vi "CDS Library Load.vi"(8 "error in (no error)":errorcluster, 11 "DMA Channel Testing in":refnum<class "DMA Channel Testing.lvclass">) -> (0 "error out":errorcluster, 3 "DMA Channel Testing out":refnum<class "DMA Channel Testing.lvclass">)   [LabVIEW 2019, in "DMA Channel Testing.lvclass"]
uses:
  DMA Channel Testing.lvclass
  DMA Channel Testing.lvclass/DMA Channel Testing.ctl
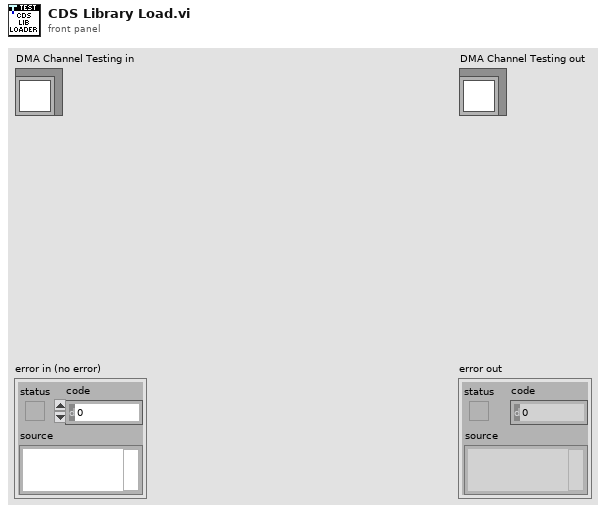
[diagram p1: front panel]
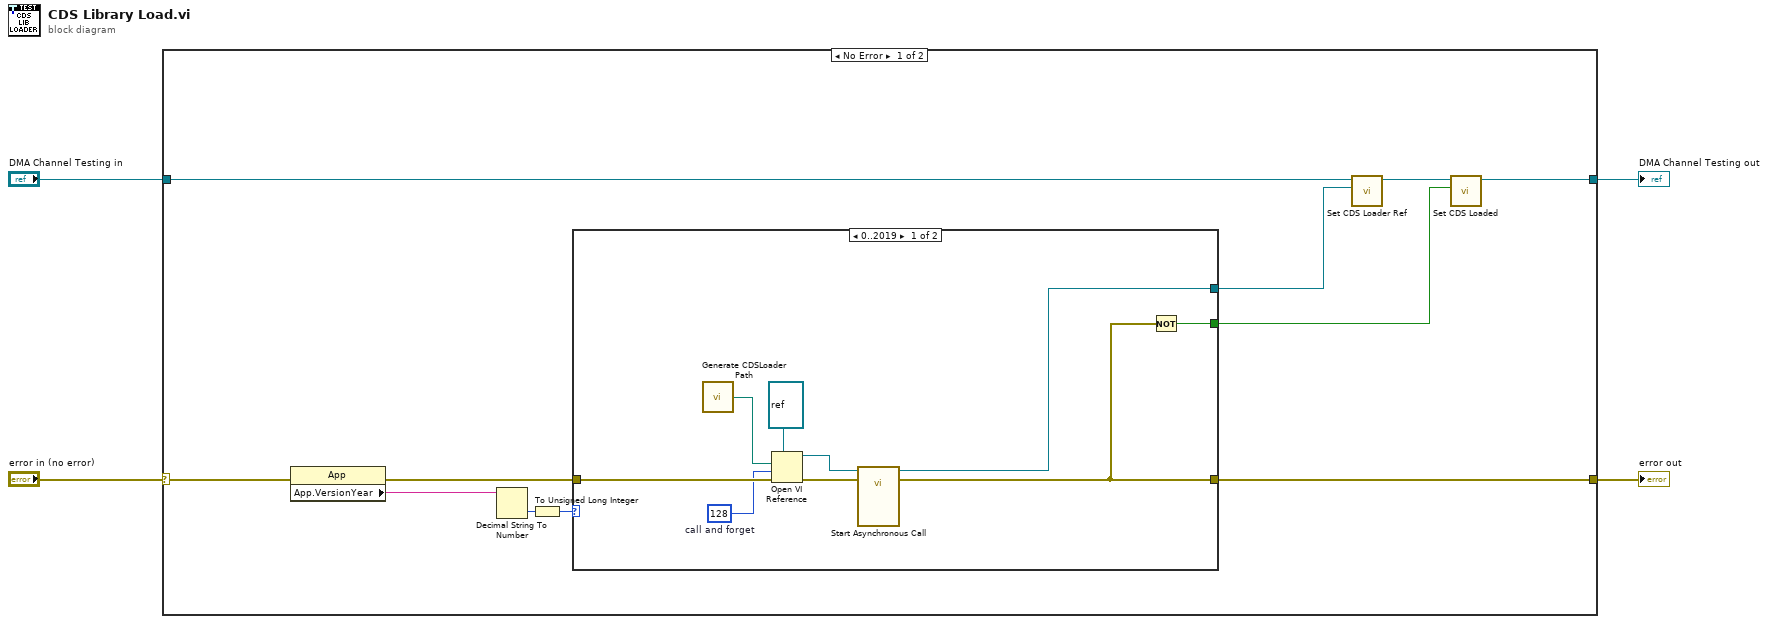
[diagram p0: block diagram]
diagram:
  n1 = case shown="No Error" "error in (no error)" {
    selector: "error in (no error)" -> [w12 w27]
    tunnel: [w10 w27] -> w3
    tunnel: [w5 w26] -> w1
    tunnel: "DMA Channel Testing in" -> [w9 w26]
    frame No Error {
      n2 = property class="App"(error in=w12) -> (error out=w11:errorcluster, "App.VersionYear"=w14:string)  [unwired: 1 in, 1 out]
      n3 = Decimal String To Number(string=w14) -> (number=w13:i32)  [unwired: 2 in, 1 out]
      n4 = To Unsigned Long Integer(number=w13) -> (unsigned 32bit integer=w15:u32)
      n5 = case shown="0..2019" w15 {
        tunnel: w11 -> [w24 w25]
        tunnel: [w17 w25] -> w10
        tunnel: [w18 _] -> w8
        tunnel: [w16 _] -> w6
        frame 0..2019 {
          w22 = 128  # call and forget
          n6 = call "Generate CDSLoader Path.vi"() -> ("CDS Loader path"=w23:path)
          n7 = Open VI Reference(type specifier VI Refnum (for type only)=refnum<vi> refnum, vi path=w23, options=w22, error in (no error)=w24) -> (vi reference=w19:refnum<vi>, error out=w20:errorcluster)  [unwired: 2 in]
          n8 = call-by-ref "Start Asynchronous Call"(reference=w19, error in=w20) -> (reference out=w18:refnum<vi>, error out=w17:errorcluster)  [unwired: 12 in]
          n9 = Not(x=w17) -> (.not. x?=w16:bool)
        }
        frame 2021.., Default {
        }
      }
      n10 = call "Set CDS Loader Ref.vi"("CDS Loader Ref"=w8, "DMA Channel Testing in"=w9) -> ("DMA Channel Testing out"=w7:refnum<class "DMA Channel Testing.lvclass">)  [unwired: 9 in]
      n11 = call "Set CDS Loaded.vi"("CDS Loaded"=w6, "DMA Channel Testing in"=w7) -> ("DMA Channel Testing out"=w5:refnum<class "DMA Channel Testing.lvclass">)  [unwired: 9 in]
    }
    frame Error {
    }
  }
  "error out" <- w3
  "DMA Channel Testing out" <- w1
